vi "Close Events.vi"(8 "Error in":errorcluster caption="Error in (no error)", 11 "Editor Events":T1) -> (0 "Error out":errorcluster)   [LabVIEW 2023, in "VIDocEditor.lvclass"]
uses:
  VIDocEditor.lvclass
  Editor Events Cluster.ctl
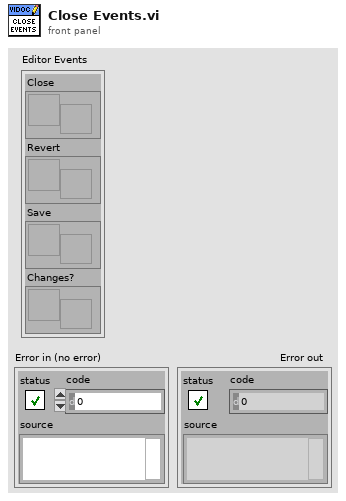
[diagram p1: front panel]
types:
  T1 = typedef "VIDocEditor.lvclass/Editor Events Cluster.ctl" = cluster{"Close":refnum<user-event>, "Revert":refnum<user-event>, "Save":refnum<user-event>, "Changes?":refnum<user-event>}
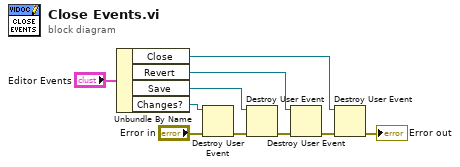
[diagram p0: block diagram]
diagram:
  n1 = Unbundle By Name("Editor Events") -> ("Close"=w1:refnum<user-event>, "Revert"=w2:refnum<user-event>, "Save"=w3:refnum<user-event>, "Changes?"=w4:refnum<user-event>)
  n2 = Destroy User Event(user event=w4, error in="Error in") -> (error out=w7:errorcluster)
  n3 = Destroy User Event(user event=w3, error in=w7) -> (error out=w6:errorcluster)
  n4 = Destroy User Event(user event=w2, error in=w6) -> (error out=w5:errorcluster)
  n5 = Destroy User Event(user event=w1, error in=w5) -> (error out=→"Error out":errorcluster)
